vi "CleanSensorArray.vi"(4 "Sensor Data Array":dbl[][](array[numeric])) -> (1 "Clean Array":dbl[][](array[numeric]))   [LabVIEW 2021]
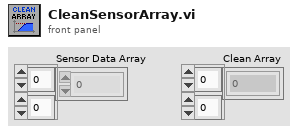
[diagram p1: front panel]
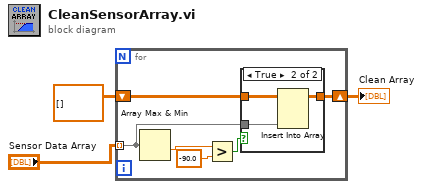
[diagram p0: block diagram]
diagram:
  n1 = for {
    tunnel: "Sensor Data Array" -> [w4] mode=indexing
    shift-right: [w8] -> w3
    shift-left: dbl[][] [] -> [w9]
    n2 = Array Max & Min(array=w4) -> (min value=w5:dbl)  [unwired: 3 out]
    n3 = Greater?(x=w5, y=-90.0) -> (0:w6:bool)
    n4 = case shown="True" w6 {
      tunnel: w9 -> [w10 w13]
      tunnel: w4 -> [_ w12]
      tunnel: [w10 w11] -> w8
      frame False {
      }
      frame True {
        n5 = Insert Into Array(array=w13, new element=w12) -> (w11:dbl[][])  [unwired: 2 in]
      }
    }
  }
  "Clean Array" <- w3
